vi "FunctDataMgr.Reference RsltTbl Controls.vi"(4 "ShowOnlyFail":refnum<vi>, 6 "AutoScroll":refnum<vi>, 7 "Filter":refnum<vi>, 8 "error in (no error)":errorcluster, 9 "Visible Rows":i32=14, 10 "RsltTbl":refnum<vi>, 11 "FunctDataMgr in":refnum<class "FunctDataMgr.lvclass">) -> (0 "error out":errorcluster, 3 "FunctDataMgr":refnum<class "FunctDataMgr.lvclass">)   [LabVIEW 2024, in "FunctDataMgr.lvclass"]
uses:
  FunctDataMgr.lvclass
  FunctDataMgr.lvclass/FunctDataMgr.ctl
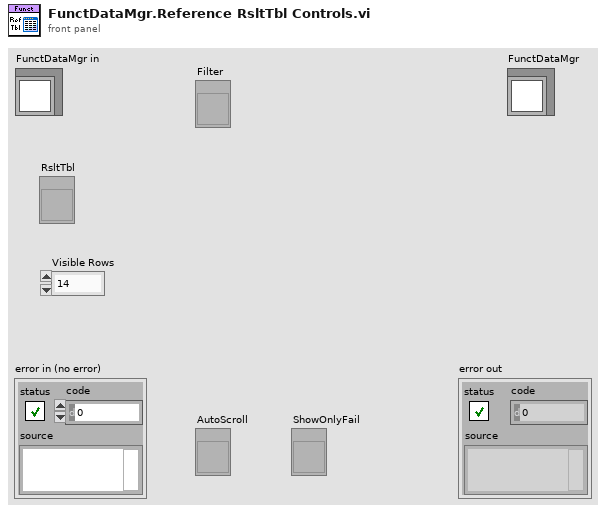
[diagram p1: front panel]
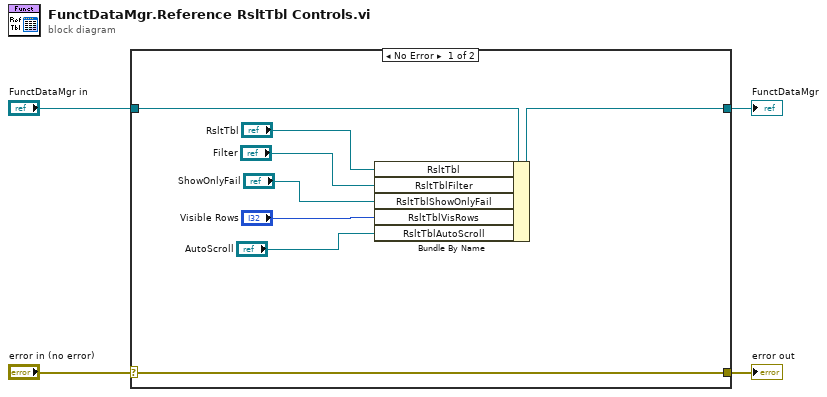
[diagram p0: block diagram]
diagram:
  n1 = case shown="No Error" "error in (no error)" {
    selector: "error in (no error)" -> [w12 w14]
    tunnel: [w12 w14] -> w3
    tunnel: [w10 w13] -> w1
    tunnel: "FunctDataMgr in" -> [w11 w13]
    frame No Error {
      n2 = Bundle By Name(cluster=w11, "RsltTbl"="RsltTbl", "RsltTblFilter"="Filter", "RsltTblShowOnlyFail"="ShowOnlyFail", "RsltTblVisRows"="Visible Rows", "RsltTblAutoScroll"="AutoScroll") -> (w10:refnum<class "FunctDataMgr.lvclass">)
    }
    frame Error {
    }
  }
  "error out" <- w3
  "FunctDataMgr" <- w1
